vi "Data Logging.vi"() -> ()   [LabVIEW 2011]
uses:
  <vilib>/Utility/file.llb/Write To Spreadsheet File (DBL).vi
panel:
  out "output array":dbl[][](array[numeric])
  out "output row":dbl[](array[numeric])
  in  "Save Data":bool
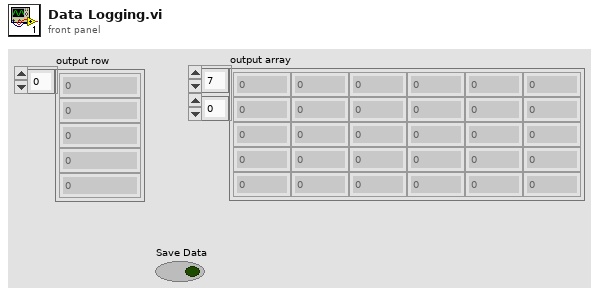
[diagram p1: front panel]
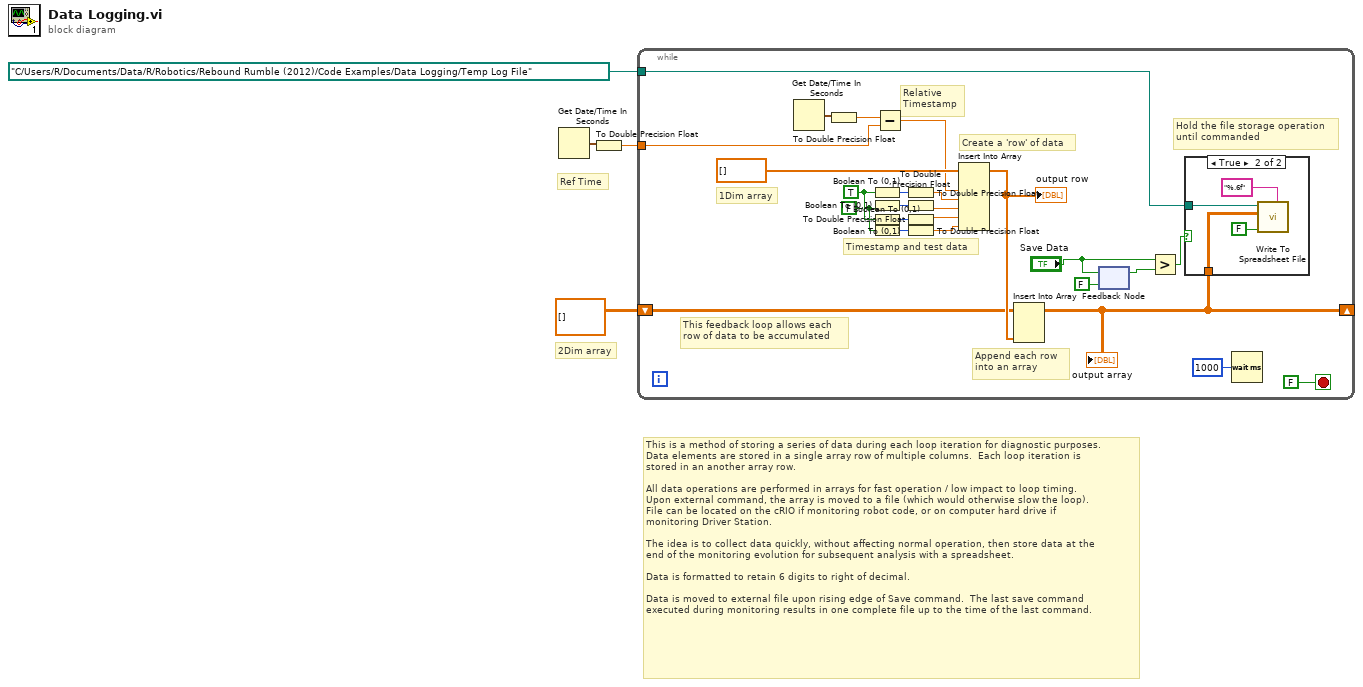
[diagram p0: block diagram]
diagram:
  # "This is a method of storing a series of data during each loop iteration for diagnostic purposes.\nData elements are stored in a single array row of multiple columns.  Each loop iteration is\nstored in an another array row.\n\nAll data operations are performed in arrays for fast operation / low impact to loop timing.\nUpon external command, the array is moved to a file (which would otherwise slow the loop).\nFile can be located on the cRIO if monitoring robot code, or on computer hard drive if \nmonitoring Driver Station.\n\nThe idea is to collect data quickly, without affecting normal operation, then store data at the \nend of the monitoring evolution for subsequent analysis with a spreadsheet.\n\nData is formatted to retain 6 digits to right of decimal.\n\nData is moved to external file upon rising edge of Save command.  The last save command\nexecuted during monitoring results in one complete file up to the time of the last command."
  # "Ref Time"
  # "2Dim array"
  n1 = Get Date/Time In Seconds() -> (seconds since 1Jan1904=w4:timestamp)
  n2 = To Double Precision Float(number=w4) -> (double precision float=w2:dbl)
  n3 = while {
    tunnel: path "C:/Users/R/Documents/Data/R/Robotics/Rebound Rumble (2012)/Code Examples/Data Logging/Temp Log File" ("datalog path (use dialog)") -> [w20]
    tunnel: w2 -> [w19]
    shift-right: [w6] -> _
    shift-left: dbl[][] [] ("array") -> [w5]
    stop <- FALSE stop-if-true
    w13 = FALSE
    w14 = TRUE ("Boolean")
    # "This feedback loop allows each\nrow of data to be accumulated"
    # "Relative\nTimestamp"
    # "1Dim array"
    # "Append each row\ninto an array"
    # "Create a 'row' of data"
    # "Timestamp and test data"
    # "Hold the file storage operation\nuntil commanded"
    n4 = Get Date/Time In Seconds() -> (seconds since 1Jan1904=w25:timestamp)
    n5 = To Double Precision Float(number=w25) -> (double precision float=w24:dbl)
    n6 = Boolean To (0,1)(Boolean=w14) -> (0, 1=w26:i16)
    n7 = Boolean To (0,1)(Boolean=w13) -> (0, 1=w27:i16)
    n8 = Boolean To (0,1)(Boolean=w14) -> (0, 1=w29:i16)
    n9 = Boolean To (0,1)(Boolean=w13) -> (0, 1=w28:i16)
    n10 = Subtract(x=w24, y=w19) -> (x-y=w16:dbl)
    n11 = To Double Precision Float(number=w26) -> (double precision float=w23:dbl)
    n12 = To Double Precision Float(number=w27) -> (double precision float=w22:dbl)
    n13 = To Double Precision Float(number=w29) -> (double precision float=w12:dbl)
    n14 = To Double Precision Float(number=w28) -> (double precision float=w15:dbl)
    n15 = Insert Into Array(array=dbl[] [], new element #1=w16, new element #2=w23, new element #3=w22, new element #4=w12, new element #5=w15) -> (w7:dbl[])  [unwired: 1 in]
    "output row" <- w7
    n16 = Insert Into Array(array=w5, new element=w7) -> (w6:dbl[][])  [unwired: 2 in]
    "output array" <- w6
    n17 = feedback-in #1("Save Data") -> ()
    n18 = feedback #1(FALSE ("Save Data")) -> (w11:bool)
    n19 = Greater?(x="Save Data", y=w11) -> (0:w8:bool)
    n20 = case shown="True" w8 {
      tunnel: w20 -> [_ w33]
      tunnel: w6 -> [_ w31]
      frame False {
      }
      frame True {
        n21 = call-poly <vilib>:"Write To Spreadsheet File.vi"("format (%.3f)"="%.6f", "append to file? (new file:F)"=FALSE, "2D data"=w31, "file path (dialog if empty)"=w33) -> ()  [unwired: 2 in, 3 out]
      }
    }
    n22 = Wait (ms)(milliseconds to wait=u32 1000) -> ()  [unwired: 1 out]
  }
